vi "channel_adapter.vi"(10 "train_sequence":cdb[](array[numeric]), 11 "Signal":cdb[](array[numeric])) -> (1 "filter_out":cdb[](array[numeric]), 2 "coe":cdb[](array[numeric]), 3 "error":dbl[](array[numeric]))   [LabVIEW 2010]
uses:
  <vilib>/addons/Modulation/Analog/controls/Complex Data Waveform.ctl
  <vilib>/addons/Adaptive Filters/NI_AdaptiveFilter.lvlib
  <vilib>/addons/Modulation/niAMT.lvlib
panel:
  in  "Signal":T1 caption="output complex waveform" {"Y" format="%.3f"; "dt" format="%^.2e"; "t0" format="%.4f"}
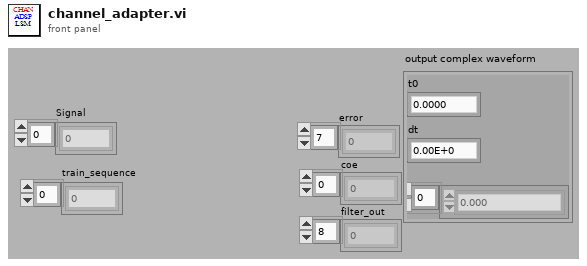
[diagram p1: front panel]
types:
  T1 = typedef "niAMT.lvlib/Complex Data Waveform.ctl" = cluster{"t0":dbl, "dt":dbl, "Y":cdb[]}
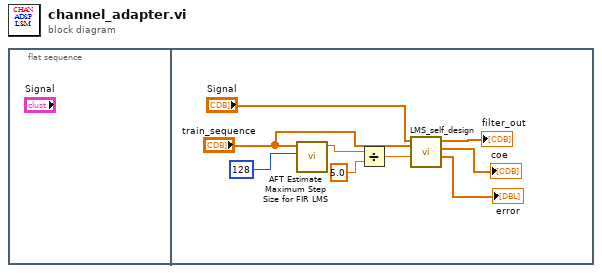
[diagram p0: block diagram]
diagram:
  n1 = flat-sequence {
    frame #0 {
    }
    frame #1 {
      n2 = call <vilib>:"AFT Estimate Maximum Step Size for FIR LMS.vi"("filter length"=128, "x(n)"="train_sequence") -> ("maximum step size"=w8:dbl)  [unwired: 8 in, 1 out]
      n3 = Divide(x=w8, y=5.0) -> (x/y=w9:dbl)
      n4 = call "LMS_self_design.vi"("step_delta"=w9, "train"="train_sequence", "sig"="Signal") -> ("error"=→"error":dbl[], "coe"=→"coe":cdb[], "filter_out"=→"filter_out":cdb[])  [unwired: 6 in]
    }
  }
